vi "Global stage boundaries.vi"() -> ()   [LabVIEW 2020]
uses:
  typedefs/typedef_boundaries.ctl
panel:
  in  "Stage boundary positions":T1={"X lower bound"=-40.0, "X upper bound"=2.6, "Y lower bound"=4.66, "Y upper bound "=12.78, "Z lower bound"=-0.001, "Z upper bound "=8.0}
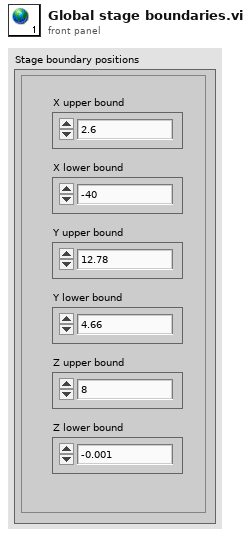
[diagram p1: front panel]
types:
  T1 = typedef "typedef_boundaries.ctl" = cluster{"X lower bound":dbl, "X upper bound":dbl, "Y lower bound":dbl, "Y upper bound ":dbl, "Z lower bound":dbl, "Z upper bound ":dbl}
diagram:
